vi "Day 04 (Part One).vi"() -> ()   [LabVIEW 2021]
uses:
  f31c8646-b681-4ab7-ad5c-a67fb4da7cfe.vi
panel:
  out "result":i32
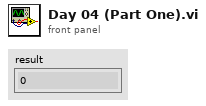
[diagram p1: front panel]
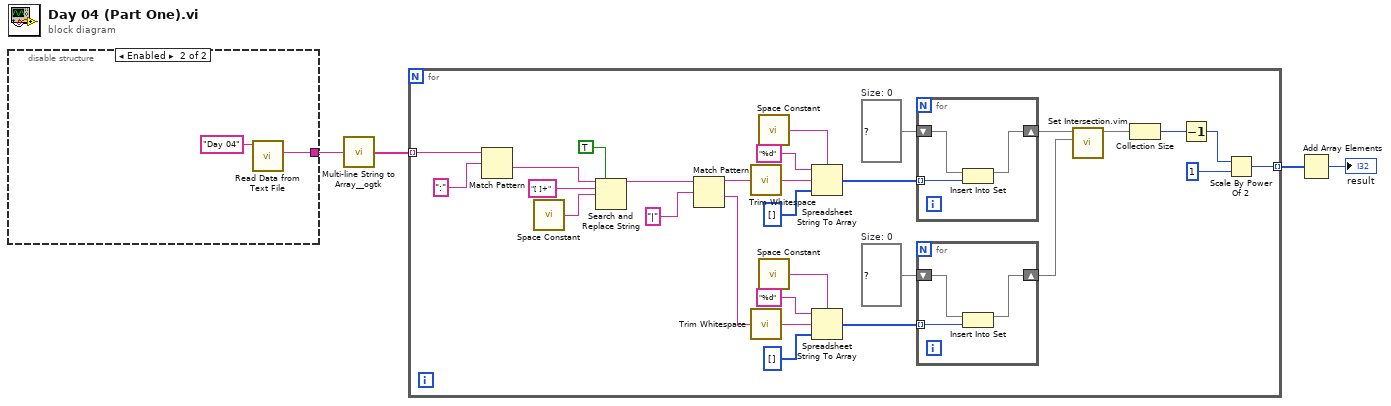
[diagram p0: block diagram]
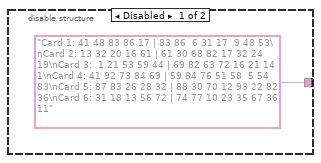
[diagram p2: hidden frame]
diagram:
  n1 = disable-structure shown="Enabled" {
    disable-tunnel: ["Card 1: 41 48 83 86 17 | 83 86  6 31 17  9 48 53\nCard 2: 13 32 20 16 61 | 61 30 68 82 17 32 24 19\nCard 3:  1 21 53 59 44 | 69 82 63 72 16 21 14  1\nCard 4: 41 92 73 84 69 | 59 84 76 51 58  5 54 83\nCard 5: 87 83 26 28 32 | 88 30 70 12 93 22 82 36\nCard 6: 31 18 13 56 72 | 74 77 10 23 35 67 36 11" w7] -> w4
    frame Disabled {
    }
    frame Enabled {
      n2 = call "Read Data from Text File.vi"("Subfolder"="Day 04") -> ("data"=w7:string)  [unwired: 10 in]
    }
  }
  n3 = call <userlib>:"Multi-line String to Array__ogtk.vi"("string"=w4) -> ("lines"=w3:string[])
  n4 = for {
    tunnel: w3 -> [w36] mode=indexing
    tunnel: [w9] -> w2 mode=indexing
    w16 = set{i32} {}  # Size: 0
    w17 = set{i32} {}  # Size: 0
    n5 = Match Pattern(string=w36, regular expression=":") -> (after substring=w23:string)  [unwired: 1 in, 3 out]
    n6 = call <vilib>:"Space Constant.vi"() -> ("String"=w20:string)
    n7 = Search and Replace String(replace all?=TRUE ("replace all? (F)"), input string=w23, search string="[ ]+", replace string=w20) -> (result string=w19:string)  [unwired: 4 in, 3 out]
    n8 = Match Pattern(string=w19, regular expression="|") -> (before substring=w27:string, after substring=w24:string)  [unwired: 1 in, 2 out]
    n9 = call <vilib>:"Trim Whitespace.vi"("string"=w27) -> ("trimmed string"=w26:string)  [unwired: 1 in]
    n10 = call <vilib>:"Trim Whitespace.vi"("string"=w24) -> ("trimmed string"=w25:string)  [unwired: 1 in]
    n11 = call <vilib>:"Space Constant.vi"() -> ("String"=w33:string)
    n12 = call <vilib>:"Space Constant.vi"() -> ("String"=w28:string)
    n13 = Spreadsheet String To Array(delimiter (Tab)=w33, format string="%d", spreadsheet string=w26, array type (2D Dbl)=i32[] []) -> (array=w18:i32[])
    n14 = Spreadsheet String To Array(delimiter (Tab)=w28, format string="%d", spreadsheet string=w25, array type (2D Dbl)=i32[] []) -> (array=w15:i32[])
    n15 = for {
      tunnel: w18 -> [w41] mode=indexing
      shift-right: [w40] -> w14
      shift-left: w17 -> [w42]
      n16 = Insert Into Set(10:w41, 11:w42) -> (3:w40:set{i32})  [unwired: 1 out]
    }
    n17 = for {
      tunnel: w15 -> [w38] mode=indexing
      shift-right: [w37] -> w13
      shift-left: w16 -> [w39]
      n18 = Insert Into Set(10:w38, 11:w39) -> (3:w37:set{i32})  [unwired: 1 out]
    }
    n19 = call "Set Intersection.vim"("set 2"=w13, "set 1"=w14) -> ("intersection"=w11:set{i32})  [unwired: 9 in]
    n20 = Collection Size(1:w11) -> (0:w10:i32)
    n21 = Decrement(x=w10) -> (x-1=w8:i32)
    n22 = Scale By Power Of 2(n=w8, x=1) -> (x*2^n=w9:i32)
  }
  n23 = Add Array Elements(numeric array=w2) -> (sum=→"result":i32)
